vi "Actor Core.vi"(8 "error in":errorcluster, 11 "RDS Controller Actor in":refnum<class "RDS Controller Actor.lvclass">) -> (0 "error out":errorcluster, 3 "Actor out":refnum<class "Actor.lvclass">)   [LabVIEW 2015, in "RDS Controller Actor.lvlib" / "RDS Controller Actor.lvclass"]
doc: "(<B>Filename</B>: Actor Framework.lvlib:Actor.lvclass:Actor Core.vi)\n\nReceives messages to the actor, reacts to them, and initiates any error handling that may shut the actor down.\n\nDescendant classes may override this VI to append parallel tasks for the actor to complete while it handles messages. Overrides use the Call Parent Method node."
uses:
  RDS Controller Actor.lvclass
  <vilib>/ActorFramework/Actor/Actor.lvclass
  <vilib>/ActorFramework/Actor/Actor.lvclass/Actor.ctl
  <vilib>/ActorFramework/Message Enqueuer/Message Enqueuer.lvclass/Message Enqueuer.ctl
  <vilib>/ActorFramework/Message Enqueuer/Init from Existing Queue.vi
  <vilib>/ActorFramework/Message Enqueuer/Message Enqueuer.lvclass
  RDS Parent Actor/RDS Parent Actor/RDS Parent Actor.lvclass
  RDS Controller Actor Messages/Controller Send State Msg/Controller Send State Msg.lvclass
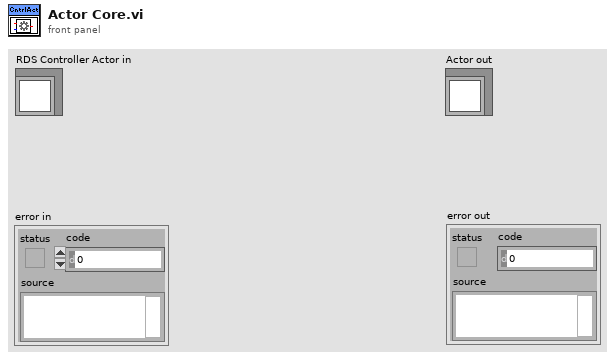
[diagram p1: front panel]
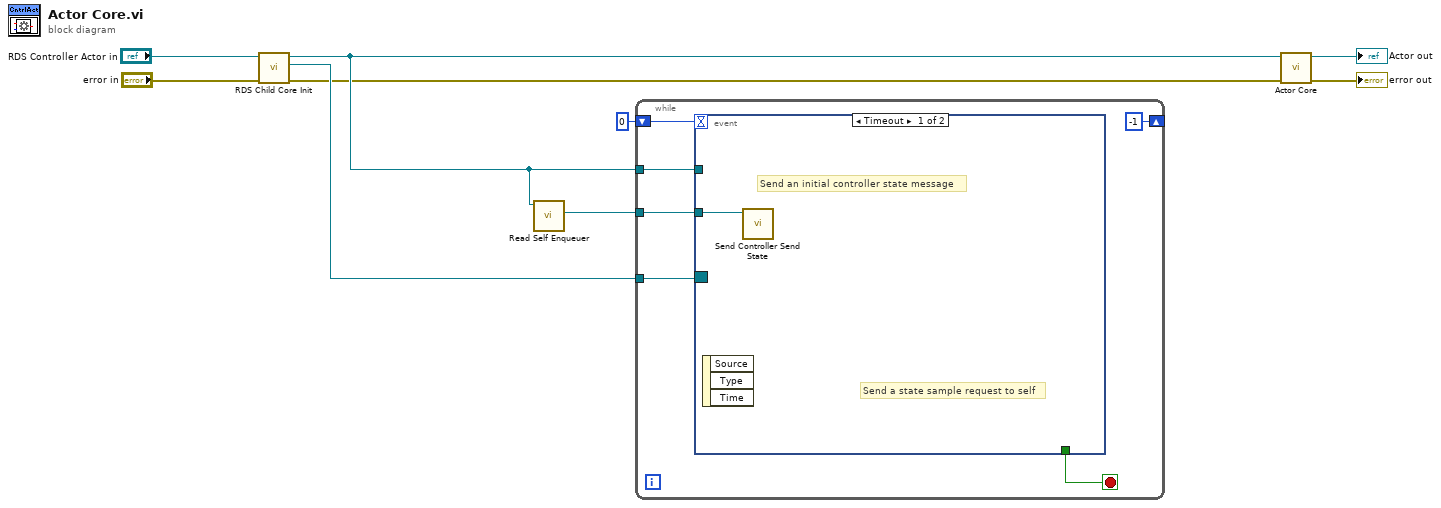
[diagram p0: block diagram]
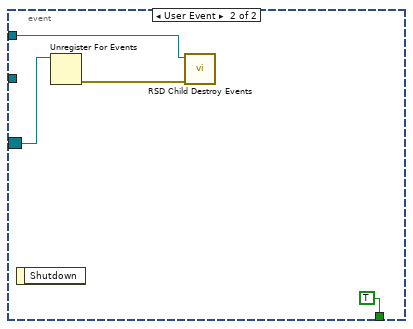
[diagram p2: hidden frame]
diagram:
  n1 = call "RDS Child Core Init.vi"("error in (no error)"="error in", "RDS Parent Actor in"="RDS Controller Actor in") -> ("error out"=w1:errorcluster, "Event Registration Refnum"=w7:refnum<event-registration>, "RDS Parent Actor out"=w3:refnum<class "RDS Controller Actor.lvclass">)  [unwired: 6 in, 1 out]
  n2 = call <vilib>:"Read Self Enqueuer.vi"("Actor"=w3) -> ("Self Enqueuer"=w2:refnum<class "Message Enqueuer.lvclass">)  [unwired: 10 in]
  n3 = while {
    tunnel: w7 -> [w14]
    tunnel: w3 -> [w15]
    shift-right: [-1] -> _
    shift-left: 0 -> [w12]
    tunnel: w2 -> [w10]
    stop <- w13 stop-if-true
    n4 = event shown="[0] Timeout" {
      selector: w14 -> [_ w18]
      dyn-events: _ -> [_ _]
      timeout: w12 -> [_ _]
      tunnel: w15 -> [_ w17]
      tunnel: [_ TRUE] -> w13
      tunnel: w10 -> [w16 _]
      event Timeout {
        # "Send an initial controller state message"
        # "Send a state sample request to self"
        n5 = event-data() -> ()  [unwired: 1 in, 3 out]
        n6 = call "Send Controller Send State.vi"("Message Enqueuer in"=w16) -> ()  [unwired: 9 in, 2 out]
      }
      event User Event {
        n7 = event-data() -> ()  [unwired: 1 in, 1 out]
        n8 = Unregister For Events(event registration refnum=w18) -> (error out=w19:errorcluster)  [unwired: 1 in]
        n9 = call "RSD Child Destroy Events.vi"("error in (no error)"=w19, "RDS Parent Actor in"=w17) -> ()  [unwired: 8 in, 2 out]
      }
    }
  }
  n10 = call-parent "Actor Core.vi"("error in"=w1, "Actor in"=w3) -> ("error out"=→"error out":errorcluster, "Actor out"=→"Actor out":refnum<class "Actor.lvclass">)  [unwired: 8 in]
